vi "Init.vi"(8 "error in (no error)":errorcluster, 9 "Meta Fields":string[](array[string])) -> (0 "error out":errorcluster, 3 "Save Filter out":refnum<class "Overlay Filter.lvclass">)   [LabVIEW 2020, in "CDM-Config.lvlib" / "Overlay Filter.lvclass"]
uses:
  Overlay Filter.lvclass
  Overlay Filter.lvclass/Overlay Filter.ctl
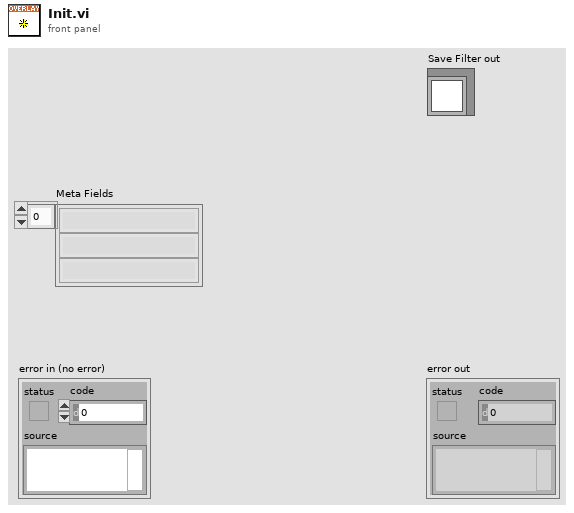
[diagram p1: front panel]
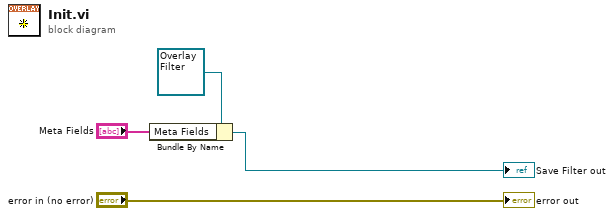
[diagram p0: block diagram]
diagram:
  n1 = Bundle By Name(cluster=refnum<class "Overlay Filter.lvclass"> refnum ("Save Filter in"), "Meta Fields"="Meta Fields") -> (→"Save Filter out":refnum<class "Overlay Filter.lvclass">)
  "error out" <- "error in (no error)"
